vi "_save_csv_HAPS_MCU_PhaseGainCali.vi"(7 "NoteName":string="SingleCh_", 9 "dup path":path, 11 "array in":string[][](array[string])) -> (3 "FileName":string)   [LabVIEW 2023, in "HAPS.lvlib"]
uses:
  HAPS.lvlib
  <vilib>/Utility/file.llb/Write Delimited Spreadsheet (string).vi
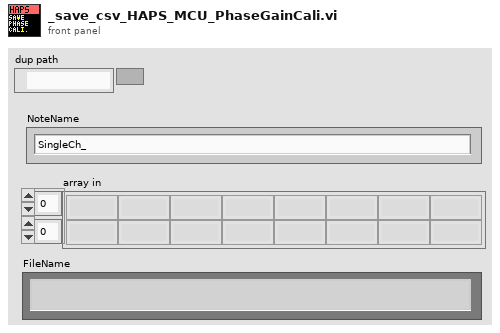
[diagram p1: front panel]
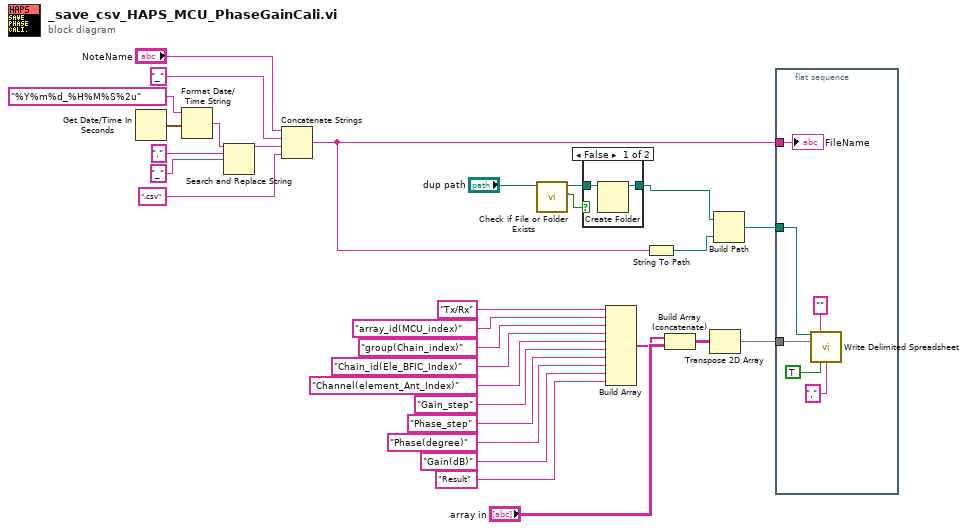
[diagram p0: block diagram]
diagram:
  n1 = Get Date/Time In Seconds() -> (seconds since 1Jan1904=w17:timestamp)
  n2 = Format Date/Time String(time format string (%c)="%Y%m%d_%H%M%S%2u", seconds (now)=w17) -> (date/time string=w15:string)  [unwired: 1 in]
  n3 = Search and Replace String(input string=w15, search string=".", replace string="_") -> (result string=w12:string)  [unwired: 5 in, 3 out]
  n4 = Concatenate Strings("NoteName", "_", w12, ".csv" ("delimiter (\\t)")) -> (w28:string)
  n5 = call <vilib>:"Check if File or Folder Exists.vi"("path"="dup path") -> ("file or folder exists?"=w4:bool, "dup path"=w3:path)  [unwired: 8 in, 1 out]
  n6 = case shown="False" w4 {
    tunnel: w3 -> [w32 w33]
    tunnel: [w31 w33] -> w1
    frame False {
      n7 = Create Folder(path (use dialog)=w32) -> (created path=w31:path)  [unwired: 2 in, 2 out]
    }
    frame True {
    }
  }
  n8 = Build Array("Tx/Rx", "array_id(MCU_index)", "group(Chain_index)", "Chain_id(Ele_BFIC_Index)", "Channel(element_Ant_Index)", "Gain_step", "Phase_step", "Phase(degree)", "Gain(dB)", "Result") -> (w20:string[])
  n9 = String To Path(string=w28) -> (path=w30:path)
  n10 = Build Array (concatenate)(w20, "array in") -> (w25:string[][])
  n11 = Transpose 2D Array(2D array=w25) -> (transposed array=w27:string[][])
  n12 = Build Path(base path=w1, name or relative path=w30) -> (appended path=w29:path)
  n13 = flat-sequence {
    tunnel: w29 -> [w38]
    tunnel: w28 -> [w36]
    tunnel: w27 -> [w34]
    frame #0 {
      n14 = call-poly <vilib>:"Write Delimited Spreadsheet.vi"("file path (dialog if empty)"=w38, "format (%s)"="" ("format (%.3f)"), "2D data"=w34, "transpose? (no:F)"=TRUE, "delimiter (\\t)"="," ("delimiter (\\t)")) -> ()  [unwired: 9 in, 2 out]
      "FileName" <- w36
    }
  }
